vi "Regulation - Interpolate and Measure.vi"(8 "error in (no error)":errorcluster, 9 "search results":cluster{"level":dbl, "value":dbl}[](array[cluster]), 10 "regulation settings":T1={"enable regulation"=FALSE, "regulation target"=enum."THD+N Ratio", "regulation target value"=0.05, "regulation target value units"=enum."%", "regulation start level"=10.0, "regulation stop level"=70.0, "regulation number of steps"=2}, 11 "measurement configuration":T5 {"acq sampling rate" format="%0.2f"; "master clock rate" format="%#_6pHz"; "frame clock rate" format="%#_6pHz"}) -> (0 "error out":errorcluster, 1 "spectrum":cluster{"x0":dbl, "dx":dbl, "magnitude":dbl[]}, 2 "time domain":waveform(dbl), 3 "results":T4, 4 "output power":dbl)   [LabVIEW 2021]
uses:
  controls/digital audio protocol/data justification.ctl
  controls/digital audio protocol/endianness.ctl
  controls/digital audio protocol/digital edge.ctl
  controls/digital audio protocol/logic level.ctl
  controls/digital output level units.ctl
  controls/weighting filter.ctl
  controls/highpass filter.ctl
  controls/lowpass filter.ctl
  controls/units - snr.ctl
  controls/units - ratio.ctl
  controls/regulation target.ctl
  controls/regulation target value units.ctl
  controls/single tone audio measurements.ctl
  <vilib>/gmath/NI_Gmath.lvlib
  controls/audio controls.lvlib
  controls/regulation settings.ctl
  controls/single tone measurement settings (HW).ctl
panel:
  out "interpolation value":dbl
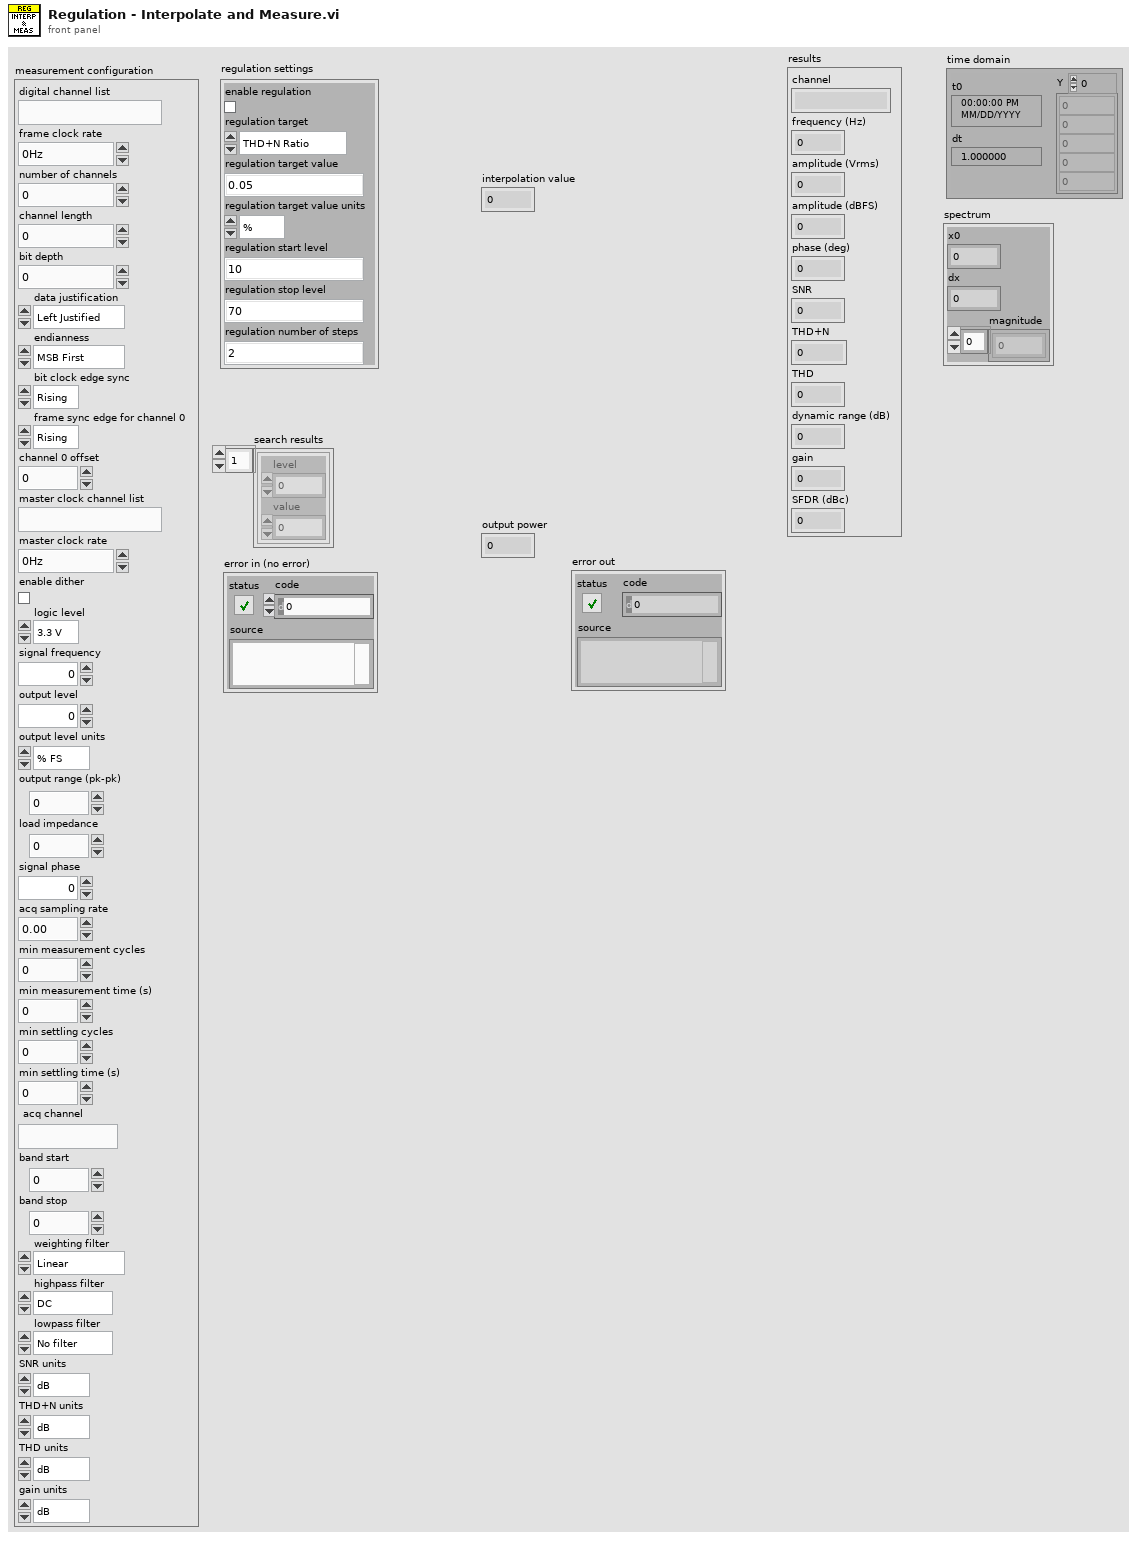
[diagram p1: front panel]
types:
  T1 = typedef "regulation settings.ctl" = cluster{"enable regulation":bool, "regulation target":T2, "regulation target value":dbl, "regulation target value units":T3, "regulation start level":dbl, "regulation stop level":dbl, "regulation number of steps":u32}
  T2 = typedef "regulation target.ctl" = enum32{"THD+N Ratio", "Output Power"}
  T3 = typedef "regulation target value units.ctl" = enum32{"%", "W"}
  T4 = typedef "audio controls.lvlib/single tone audio measurements.ctl" = cluster{"channel":string, "frequency (Hz)":dbl, "amplitude (Vrms)":dbl, "amplitude (dBFS)":dbl, "phase (deg)":dbl, "SNR":dbl, "THD+N":dbl, "THD":dbl, "dynamic range (dB)":dbl, "gain":dbl, "SFDR (dBc)":dbl}
  T5 = typedef "single tone measurement settings (HW).ctl" = cluster{"digital channel list":string, "frame clock rate":dbl, "number of channels":u32, "channel length":u32, "bit depth":u32, "data justification":T6, "endianness":T7, "bit clock edge sync":T8, "frame sync edge for channel 0":T8, "channel 0 offset":u32, "master clock channel list":string, "master clock rate":dbl, "enable dither":bool, "logic level":T9, "signal frequency":dbl, "output level":dbl, "output level units":T10, "output range (pk-pk)":dbl, "load impedance":dbl, "signal phase":dbl, "acq sampling rate":dbl, "min measurement cycles":u32, "min measurement time (s)":dbl, "min settling cycles":u32, "min settling time (s)":dbl, "acq channel":string, "band start":dbl, "band stop":dbl, "weighting filter":T11, "highpass filter":T12, "lowpass filter":T13, "SNR units":T14, "THD+N units":T15, "THD units":T15, "gain units":T15}
  T6 = typedef "data justification.ctl" = enum32{"Left Justified", "Right Justified"}
  T7 = typedef "endianness.ctl" = enum32{"MSB First", "LSB First"}
  T8 = typedef "digital edge.ctl" = enum32{"Rising", "Falling"}
  T9 = typedef "logic level.ctl" = enum32{"3.3 V", "1.8 V", "1.2 V"}
  T10 = typedef "audio controls.lvlib/digital output level units.ctl" = enum32{"% FS", "dBFS"}
  T11 = typedef "weighting filter.ctl" = enum32{"Linear", "A-weighting", "B-weighting", "C-weighting"}
  T12 = typedef "highpass filter.ctl" = enum32{"DC", "AC"}
  T13 = typedef "lowpass filter.ctl" = enum32{"No filter", "AES17 20kHz", "AES17 40kHz"}
  T14 = typedef "audio controls.lvlib/units - snr.ctl" = enum32{"dB", "x/y"}
  T15 = typedef "audio controls.lvlib/units - ratio.ctl" = enum32{"dB", "%", "x/y"}
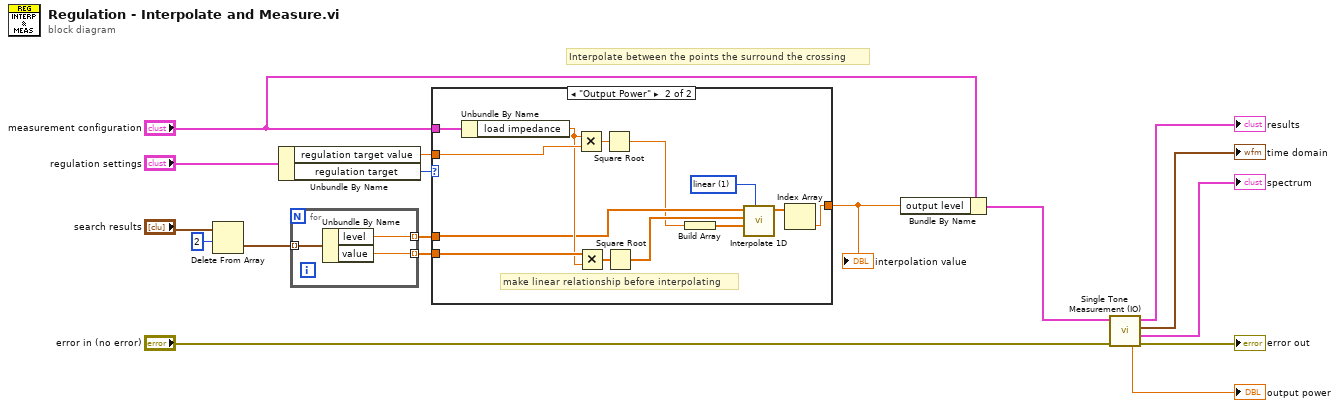
[diagram p0: block diagram]
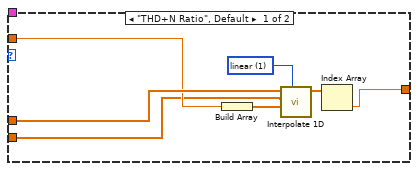
[diagram p2: hidden frame]
diagram:
  # "Interpolate between the points the surround the crossing"
  n1 = Delete From Array(array="search results", length=2) -> (deleted portion=w2:cluster{"level":dbl, "value":dbl}[])  [unwired: 1 in, 1 out]
  n2 = Unbundle By Name("regulation settings") -> ("regulation target value"=w13:dbl, "regulation target"=w7:T2)
  n3 = for {
    tunnel: w2 -> [w20] mode=indexing
    tunnel: [w19] -> w5 mode=indexing
    tunnel: [w18] -> w6 mode=indexing
    n4 = Unbundle By Name(w20) -> ("level"=w18:dbl, "value"=w19:dbl)
  }
  n5 = case shown="\"Output Power\"" w7 {
    tunnel: w13 -> [w23 w36]
    tunnel: [w25 w28] -> w12
    tunnel: w6 -> [w24 w34]
    tunnel: w5 -> [w21 w37]
    tunnel: "measurement configuration" -> [_ w40]
    frame "THD+N Ratio", Default {
      w27 = 1 items=["nearest", "linear", "spline", "cubic Hermite", "Lagrange"] ("method")
      n6 = Build Array(w23) -> (w22:dbl[])
      n7 = call <vilib>:"Interpolate 1D.vi"("method"=w27, "xi"=w22, "X"=w21, "Y"=w24) -> ("yi"=w26:dbl[])  [unwired: 5 in, 2 out]
      n8 = Index Array(array=w26) -> (element=w25:dbl)  [unwired: 1 in]
    }
    frame "Output Power" {
      w30 = 1 items=["nearest", "linear", "spline", "cubic Hermite", "Lagrange"] ("method")
      # "make linear relationship before interpolating"
      n9 = Unbundle By Name(w40) -> ("load impedance"=w35:dbl)
      n10 = Multiply(x=w35, y=w36) -> (x*y=w39:dbl)
      n11 = Multiply(x=w37, y=w35) -> (x*y=w38:dbl[])
      n12 = Square Root(x=w39) -> (sqrt(x)=w32:dbl)
      n13 = Square Root(x=w38) -> (sqrt(x)=w33:dbl[])
      n14 = Build Array(w32) -> (w31:dbl[])
      n15 = call <vilib>:"Interpolate 1D.vi"("method"=w30, "xi"=w31, "X"=w33, "Y"=w34) -> ("yi"=w29:dbl[])  [unwired: 5 in, 2 out]
      n16 = Index Array(array=w29) -> (element=w28:dbl)  [unwired: 1 in]
    }
  }
  "interpolation value" <- w12
  n17 = Bundle By Name(cluster="measurement configuration", "output level"=w12) -> (w15:T5)
  n18 = call "Single Tone Measurement (IO).vi"("error in (no error)"="error in (no error)", "measurement configuration"=w15) -> ("error out"=→"error out":errorcluster, "spectrum"=→"spectrum":cluster{"x0":dbl, "dx":dbl, "magnitude":dbl[]}, "time domain"=→"time domain":waveform(dbl), "results"=→"results":T4, "output power"=→"output power":dbl)  [unwired: 5 in]
